vi "Sound-Get Input Device By Name.vi"(7 "Name":string) -> (8 "Audio Device Info":T1, 15 "error out":errorcluster)   [LabVIEW 2020]
uses:
  <vilib>/Dataflow_G/G-Audio/Controls/Audio Device Info.ctl
  <vilib>/Dataflow_G/G-Audio/Controls/Audio Device Type.ctl
  <vilib>/Dataflow_G/G-Audio/Controls/Audio Device Native Data Format.ctl
  <vilib>/Dataflow_G/G-Audio/Controls/Audio Device Format.ctl
  <vilib>/Utility/error.llb/Error Cluster From Error Code.vi
  <vilib>/ErrorRing/Error Ring.xnode
  <vilib>/Dataflow_G/G-Audio/G-Audio.lvlib
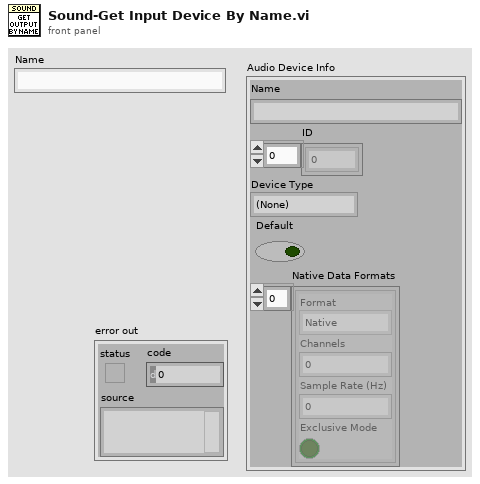
[diagram p1: front panel]
types:
  T1 = typedef "G-Audio.lvlib/Audio Device Info.ctl" = cluster{"Name":string, "ID":u8[], "Device Type":T2, "Default":bool, "Native Data Formats":T3[]}
  T2 = typedef "G-Audio.lvlib/Audio Device Type.ctl" = enum16{"(None)", "Playback", "Capture", "Duplex", "Loopback"}
  T3 = typedef "G-Audio.lvlib/Audio Device Native Data Format.ctl" = cluster{"Format":T4, "Channels":u32, "Sample Rate (Hz)":u32, "Exclusive Mode":bool}
  T4 = typedef "G-Audio.lvlib/Audio Device Format.ctl" = enum16{"Native", "U8", "I16", "I32", "SGL"}
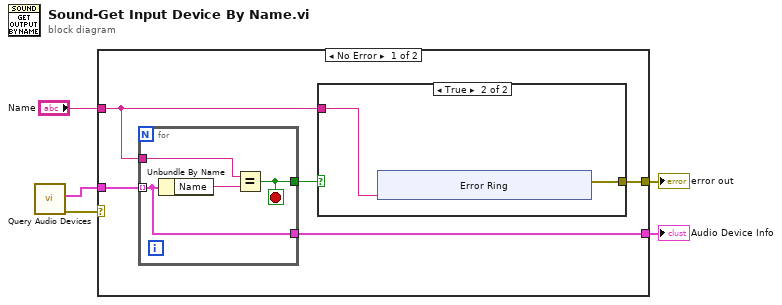
[diagram p0: block diagram]
diagram:
  n1 = call <vilib>:"Query Audio Devices.vi"() -> ("error out"=w4:errorcluster, "Capture Devices"=w1:T1[])  [unwired: 7 in, 3 out]
  n2 = case shown="No Error" w4 {
    selector: w4 -> [_ w24]
    tunnel: w1 -> [w10 _]
    tunnel: "Name" -> [w6 _]
    tunnel: [w8 _] -> w3
    tunnel: [w7 w24] -> w2
    frame No Error {
      n3 = for {
        tunnel: w10 -> [w23] mode=indexing
        tunnel: [w23] -> w8
        tunnel: w6 -> [w22]
        tunnel: [w20] -> w9
        stop <- w20 stop-if-true
        n4 = Unbundle By Name(w23) -> ("Name"=w21:string)
        n5 = Equal?(x=w22, y=w21) -> (x = y?=w20:bool)
      }
      n6 = case shown="True" w9 {
        tunnel: [_ w12] -> w7
        tunnel: w6 -> [_ w11]
        frame False {
        }
        frame True {
          n7 = xnode "Error Ring"("parameter 0"=w11) -> ("error out"=w12:errorcluster)
        }
      }
    }
    frame Error {
    }
  }
  "error out" <- w2
  "Audio Device Info" <- w3
